vi "motorPosControl (SubVI).vi"(6 "Reset":bool, 7 "+/- Range":dbl, 8 "error in (no error)":errorcluster, 9 "PID gains":T1={"proportional gain (Kc)"=2.0, "integral time (Ti, min)"=0.01, "derivative time (Td, min)"=0.00010000000000000003}, 10 "Position (deg)":dbl) -> (0 "error out":errorcluster, 1 "Waveform Chart":T2(graph), 2 "MotorEncoder (deg)":dbl, 4 "out of range!":bool)   [LabVIEW 2019, in "SJCube_ElvisIII.lvlib"]
uses:
  SJCube_ElvisIII.lvlib
  <vilib>/addons/control/pid/pid.llb/PID (DBL).vi
  <vilib>/addons/control/pid/NI_PID_pid.lvlib
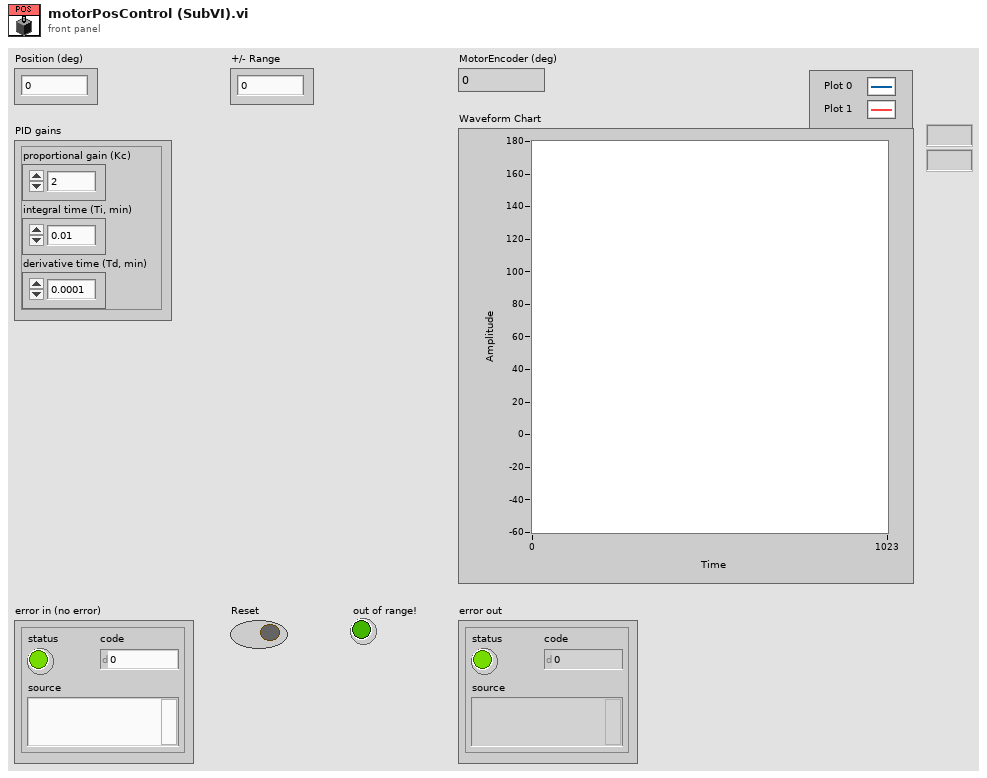
[diagram p1: front panel]
types:
  T1 = cluster{"proportional gain (Kc)":dbl, "integral time (Ti, min)":dbl, "derivative time (Td, min)":dbl}
  T2 = cluster{"Position (deg)":dbl, "MotorEncoder (deg)":dbl}
  T3 = cluster{"+/- Range":dbl, "MotorEncoder (deg)":dbl}
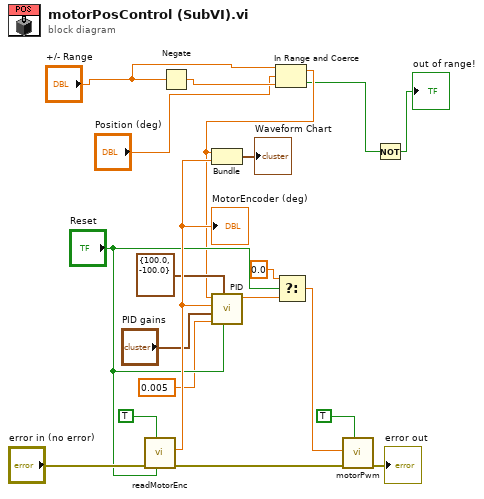
[diagram p0: block diagram]
diagram:
  n1 = call "readMotorEnc.vi"("Reset Counter"="Reset", "Reverse ENC?"=TRUE, "error in (no error)"="error in (no error)") -> ("error out"=w12:errorcluster, "MotorEncoder (deg)"=w18:dbl)  [unwired: 7 in]
  "MotorEncoder (deg)" <- w18
  n2 = Negate(x="+/- Range") -> (-x=w6:dbl)
  n3 = In Range and Coerce(upper limit="+/- Range", x="Position (deg)", lower limit=w6) -> (coerced(x)=w3:dbl, In Range?=w2:bool)
  n4 = Bundle("+/- Range"=w3, "MotorEncoder (deg)"=w18) -> (→"Waveform Chart":T3)  [unwired: 1 in]
  n5 = call-poly <vilib>:"PID.vi"("reinitialize? (F)"="Reset", "output range"=cluster{"output high":dbl, "output low":dbl} {"output high"=100.0, "output low"=-100.0}, "dt (s)"=0.005, "PID gains"="PID gains", "process variable"=w18, "setpoint"=w3) -> ("output"=w16:dbl)  [unwired: 4 in, 1 out]
  n6 = Select(t=0.0, s="Reset", f=w16) -> (s? t:f=w17:dbl)
  n7 = call "motorPwm.vi"("reverse?"=TRUE, "error in (no error)"=w12, "Speed (PWM)"=w17) -> ("error out"=→"error out":errorcluster)  [unwired: 8 in]
  n8 = Not(x=w2) -> (.not. x?=→"out of range!":bool)
